vi "Image Display Get ROI Characteristics.vi"(6 "ROI Characteristics Selection":T1={"Area (pixels)"=TRUE, "% of Image"=TRUE, "Total Intensity"=TRUE, "Mean Intensity"=TRUE, "Median Intensity"=TRUE, "Mode Intensity"=TRUE, "Intensity Standard Deviation"=TRUE, "Min Intensity"=TRUE, "Max Intensity"=TRUE, "Mean SNR"=TRUE, "Median SNR"=TRUE, "Mode SNR"=TRUE, "SNR Standard Deviation"=TRUE, "Max SNR"=TRUE, "Min SNR"=TRUE, "# Rejected Pixels (NaN, Inf)"=TRUE, "# Negative Pixels"=TRUE, "Long Axis Length"=FALSE, "Short Axis Length"=FALSE, "Aspect Ratio"=FALSE}, 8 "Error In":errorcluster, 9 "ROI Mask refnum":T4, 10 "Image refnum":T4, 11 "Image Control Refnum":T5) -> (0 "Error Out":errorcluster, 1 "ROI":T3, 2 "ROI Characteristics String":string, 3 "ROI Characteristics":T2)   [LabVIEW 2021, in "Image.lvlib"]
uses:
  Image.lvlib
  Image Control Refnum.ctl
  <vilib>/vision/Image Controls.llb/IMAQ Image.ctl
  Image ROI Statistics.ctl
  Image ROI Statistics Selection.ctl
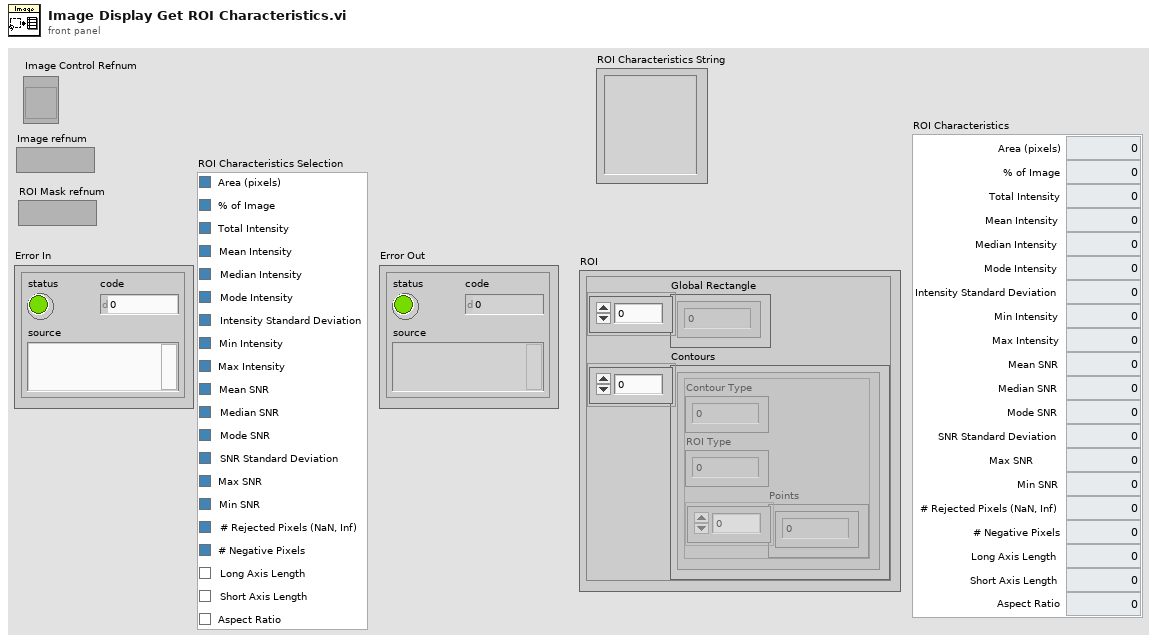
[diagram p1: front panel]
types:
  T1 = typedef "Image.lvlib/Image ROI Statistics Selection.ctl" = cluster{"Area (pixels)":bool, "% of Image":bool, "Total Intensity":bool, "Mean Intensity":bool, "Median Intensity":bool, "Mode Intensity":bool, "Intensity Standard Deviation":bool, "Min Intensity":bool, "Max Intensity":bool, "Mean SNR":bool, "Median SNR":bool, "Mode SNR":bool, "SNR Standard Deviation":bool, "Max SNR":bool, "Min SNR":bool, "# Rejected Pixels (NaN, Inf)":bool, "# Negative Pixels":bool, "Long Axis Length":bool, "Short Axis Length":bool, "Aspect Ratio":bool}
  T2 = typedef "Image.lvlib/Image ROI Statistics.ctl" = cluster{"Area (pixels)":dbl, "% of Image":dbl, "Total Intensity":dbl, "Mean Intensity":dbl, "Median Intensity":dbl, "Mode Intensity":dbl, "Intensity Standard Deviation":dbl, "Min Intensity":dbl, "Max Intensity":dbl, "Mean SNR":dbl, "Median SNR":dbl, "Mode SNR":dbl, "SNR Standard Deviation":dbl, "Max SNR":dbl, "Min SNR":dbl, "# Rejected Pixels (NaN, Inf)":dbl, "# Negative Pixels":dbl, "Long Axis Length":dbl, "Short Axis Length":dbl, "Aspect Ratio":dbl}
  T3 = cluster{"Global Rectangle":i32[], "Contours":cluster{"Contour Type":u32, "ROI Type":u32, "Points":i32[]}[]}
  T4 = typedef "IMAQ Image.ctl" = refnum<image>
  T5 = typedef "Image.lvlib/Image Control Refnum.ctl" = refnum<vi>
  T6 = cluster{"Global Rectangle":i32[], "Contours":cluster{"Contour Type":u32, "ROI Type":u32, "Points":i32[]}[]}[]
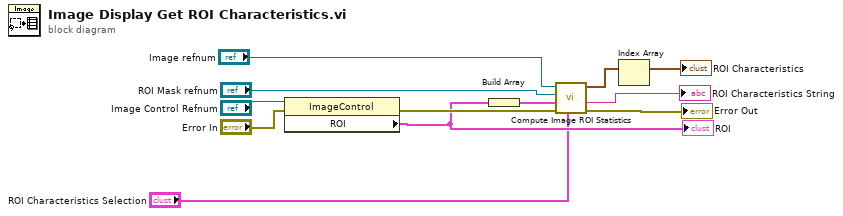
[diagram p0: block diagram]
diagram:
  n1 = property class="ImageControl"(reference="Image Control Refnum", error in="Error In") -> (error out=w10:errorcluster, "ROI"=w4:T3)  [unwired: 1 out]
  "ROI" <- w4
  n2 = Build Array(w4) -> (w3:T6)
  n3 = call "Compute Image ROI Statistics.vi"("ROI Characteristics Selection"="ROI Characteristics Selection", "error in (no error)"=w10, "ROIs"=w3, "ROI Mask Refnum"="ROI Mask refnum", "Image Refnum"="Image refnum") -> ("error out"=→"Error Out":errorcluster, "ROI Characteristics String"=→"ROI Characteristics String":string, "ROI Characteristics"=w5:T2[])  [unwired: 4 in]
  n4 = Index Array(array=w5) -> (element=→"ROI Characteristics":T2)  [unwired: 1 in]
